vi "write_to_test_params.vi"(0 "error out":errorcluster, 8 "error in (no error)":errorcluster, 10 "New_time_stamp":string, 11 "file path (dialog if empty)":path) -> ()   [LabVIEW 2018]
uses:
  SupportVIs/Read Delimited Spreadsheet (string).vi
  SupportVIs/Write Delimited Spreadsheet (string).vi
panel:
  out "all rows":string[][](array[string])
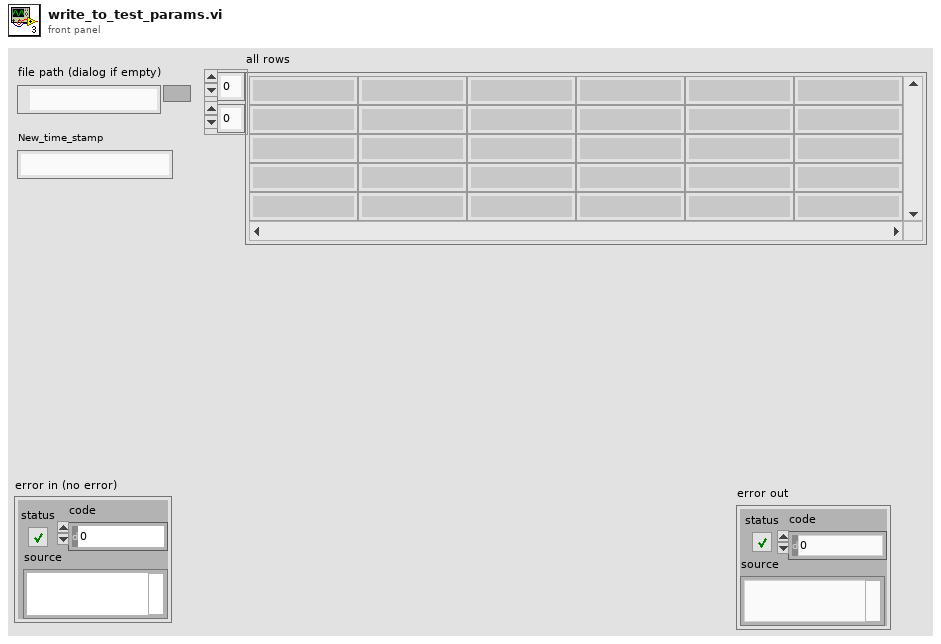
[diagram p1: front panel]
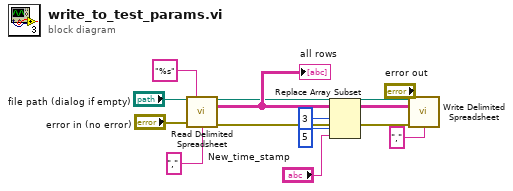
[diagram p0: block diagram]
diagram:
  n1 = call-poly "Read Delimited Spreadsheet.vi"("file path (dialog if empty)"="file path (dialog if empty)", "format (%s)"="%s", "error in (no error)"="error in (no error)", "delimiter (\\t)"="," ("delimiter (\\t)")) -> ("new file path (Not A Path if cancelled)"=w4:path, "all rows"=w8:string[][], "error out"=w2:errorcluster)  [unwired: 6 in, 3 out]
  "all rows" <- w8
  n2 = Replace Array Subset(array=w8, new element="New_time_stamp", index (row)=3, index (col)=5 ("disabled index (col)")) -> (w3:string[][])
  n3 = call-poly "Write Delimited Spreadsheet.vi"("file path (dialog if empty)"=w4, "2D data"=w3, "error in (no error)"=w2, "delimiter (\\t)"="," ("delimiter (\\t)")) -> ()  [unwired: 10 in, 2 out]
